vi "Read.vi"(5 "Timeout (1000 ms)":u16=1000, 7 "I2C Channel":u8, 8 "Error In":errorcluster, 11 "LINX Resource":T1) -> (0 "Error Out":errorcluster, 2 "Time Stamp":timestamp, 3 "LINX Resource":T1)   [LabVIEW 2013, in "LVH-LINX.lvlib" / "DS1307.lvlib"]
doc: "Read time from DS1307."
uses:
  DS1307.lvlib
  LVH-LINX.lvlib
  <vilib>/LabVIEW Hacker/LVH-Toolbox/Common/LVH-Common.lvlib
  <vilib>/Utility/miscctls.llb/LVDateTimeRec.ctl
  Private/Type Defs/Platform.ctl
  Private/Type Defs/Interface.ctl
  Private/Device/Type Defs/TCP Config.ctl
  Private/Device/Device.lvlib
  Private/Type Defs/Device Family.ctl
  Private/Device/Type Defs/LINX Device Config.ctl
  Private/Type Defs/LINX Ref.ctl
  Private/Device/Type Defs/Channels.ctl
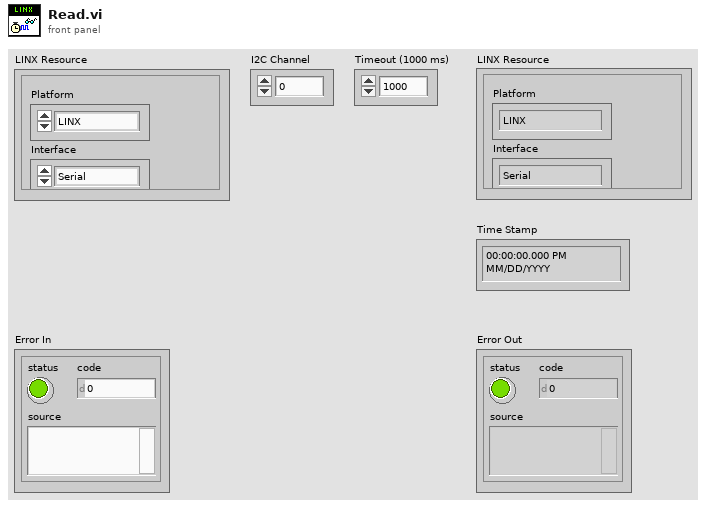
[diagram p1: front panel]
types:
  T1 = typedef "LVH-LINX.lvlib/LINX Ref.ctl" = cluster{"Platform":T2, "Interface":T3, "LINX Device Config":T4}
  T2 = typedef "LVH-LINX.lvlib/Platform.ctl" = enum16{"LINX", "myRIO"}
  T3 = typedef "LVH-LINX.lvlib/Interface.ctl" = enum16{"Serial", "TCP"}
  T4 = typedef "LVH-LINX.lvlib/Device.lvlib/LINX Device Config.ctl" = cluster{"Interface":T3, "COM Port":refnum<visa-resource-name>, "TCP Configuration":T5, "Device Family":T6, "Device ID":u8, "Device Name":string, "TCP Ref":refnum<k5>, "Channels":T7}
  T5 = typedef "LVH-LINX.lvlib/Device.lvlib/TCP Config.ctl" = cluster{"IP Address":string, "Port":u16}
  T6 = typedef "LVH-LINX.lvlib/Device Family.ctl" = enum8{"National Instruments", "Digilent", "Arduino"}
  T7 = typedef "LVH-LINX.lvlib/Channels.ctl" = cluster{"DI Channels":u8[], "DO Channels":u8[], "AI":u8[], "AO":u8[], "PWM":u8[], "QE":u8[], "UART":u8[], "I2C 2":u8[], "SPI":u8[], "CAN":u8[], "AI Ref (V)":dbl, "AO Resolution (Bits)":u8, "AO Ref (V)":dbl}
  T8 = typedef "LVDateTimeRec.ctl" = cluster{"fractional second":dbl, "second":i32, "minute":i32, "hour":i32, "day of month":i32, "month":i32, "year":i32, "day of week":i32, "day of year":i32, "DST":i32}
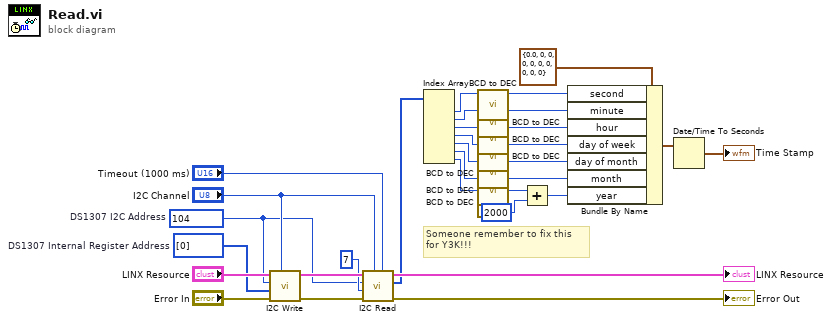
[diagram p0: block diagram]
diagram:
  w23 = u8[] [0]  # DS1307 Internal Register Address
  w21 = u8 104  # DS1307 I2C Address
  # "Someone remember to fix this \nfor Y3K!!!"
  n1 = call "I2C Write.vi"("I2C Channel"="I2C Channel", "Error In"="Error In", "Data"=w23, "I2C Slave Address (0)"=w21, "LINX Resource"="LINX Resource") -> ("Error Out"=w30:errorcluster, "LINX Resource"=w31:T1)  [unwired: 5 in]
  n2 = call "I2C Read.vi"("Timeout (1000 ms)"="Timeout (1000 ms)", "I2C Channel"="I2C Channel", "Error In"=w30, "Bytes To Read"=u8 7, "I2C Slave Address (0)"=w21, "LINX Resource"=w31) -> ("Error Out"=→"Error Out":errorcluster, "Data"=w17:u8[], "LINX Resource"=→"LINX Resource":T1)  [unwired: 3 in]
  n3 = Index Array(array=w17) -> (element #1=w20:u8, element #2=w19:u8, element #3=w18:u8, element #4=w11:u8, element #5=w10:u8, element #6=w9:u8, element #7=w8:u8)  [unwired: 7 in]
  n4 = call <vilib>:"BCD to DEC.vi"("BCD"=w20) -> ("DEC"=w14:u16)  [unwired: 10 in]
  n5 = call <vilib>:"BCD to DEC.vi"("BCD"=w19) -> ("DEC"=w13:u16)  [unwired: 10 in]
  n6 = call <vilib>:"BCD to DEC.vi"("BCD"=w18) -> ("DEC"=w12:u16)  [unwired: 10 in]
  n7 = call <vilib>:"BCD to DEC.vi"("BCD"=w11) -> ("DEC"=w4:u16)  [unwired: 10 in]
  n8 = call <vilib>:"BCD to DEC.vi"("BCD"=w10) -> ("DEC"=w5:u16)  [unwired: 10 in]
  n9 = call <vilib>:"BCD to DEC.vi"("BCD"=w9) -> ("DEC"=w6:u16)  [unwired: 10 in]
  n10 = call <vilib>:"BCD to DEC.vi"("BCD"=w8) -> ("DEC"=w7:u16)  [unwired: 10 in]
  n11 = Add(x=w7, y=u16 2000) -> (x+y=w15:u16)
  n12 = Bundle By Name(cluster=T8 {"fractional second"=0.0, "second"=0, "minute"=0, "hour"=0, "day of month"=0, "month"=0, "year"=0, "day of week"=0, "day of year"=0, "DST"=0} ("date time rec"), "second"=w14, "minute"=w13, "hour"=w12, "day of week"=w4, "day of month"=w5, "month"=w6, "year"=w15) -> (w3:T8)
  n13 = Date/Time To Seconds(2:w3) -> (0:→"Time Stamp":timestamp)  [unwired: 1 in]
